vi "Day 20-Add Padding3.vi"(10 "Padding Value":bool, 11 "Array in":bool[][](array[boolean])) -> (3 "Array out":bool[][](array[boolean]))   [LabVIEW 2021]
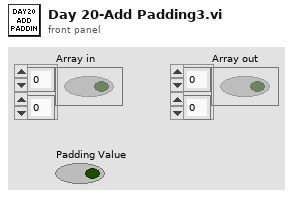
[diagram p1: front panel]
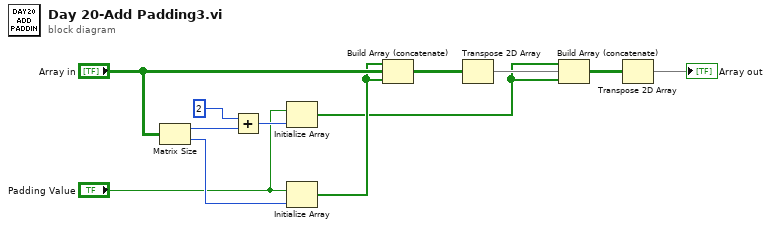
[diagram p0: block diagram]
diagram:
  n1 = Matrix Size(0:"Array in") -> (1:w9:i32, 2:w12:i32)
  n2 = Add(x=2, y=w9) -> (x+y=w7:i32)
  n3 = Initialize Array("Padding Value", w7) -> (w2:bool[])
  n4 = Initialize Array("Padding Value", w12) -> (w10:bool[])
  n5 = Build Array (concatenate)(w10, "Array in", w10) -> (w5:bool[][])
  n6 = Transpose 2D Array(2D array=w5) -> (transposed array=w4:bool[][])
  n7 = Build Array (concatenate)(w2, w4, w2) -> (w3:bool[][])
  n8 = Transpose 2D Array(2D array=w3) -> (transposed array=→"Array out":bool[][])
